vi "Alarm_TC_Cat.vi"() -> ()   [LabVIEW 2014]
panel:
  in  "T Target":dbl
  out "Error":u32
  in  "T Stoic":dbl
  out "Status Out":i32=300
  in  "Status In":i32=300
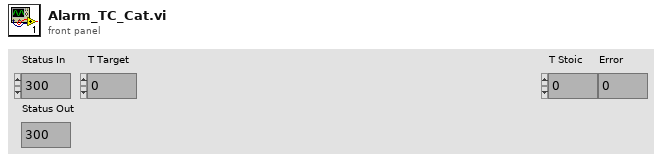
[diagram p1: front panel]
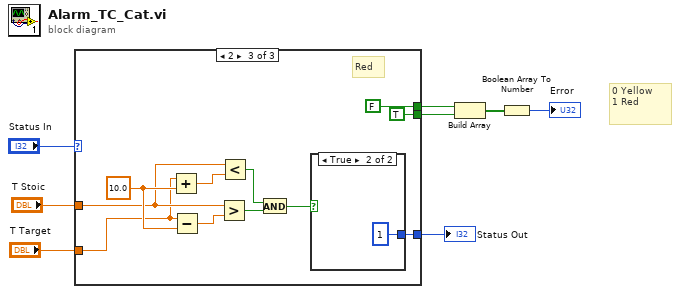
[diagram p0: block diagram]
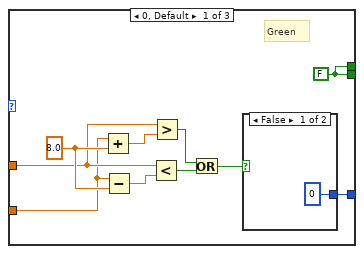
[diagram p2: hidden frame]
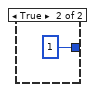
[diagram p3: hidden frame]
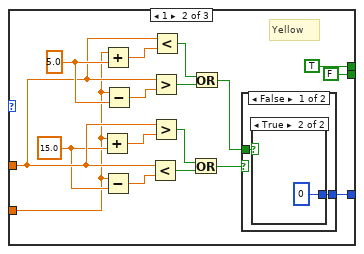
[diagram p4: hidden frame]
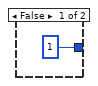
[diagram p5: hidden frame]
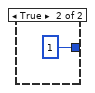
[diagram p6: hidden frame]
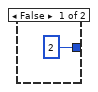
[diagram p7: hidden frame]
diagram:
  # "0 Yellow\n1 Red"
  n1 = case shown="2" "Status In" {
    tunnel: "T Stoic" -> [w11 w24 w47]
    tunnel: [w15 w32 w46] -> w6
    tunnel: [w10 TRUE ("x .or. y?") FALSE ("x .or. y?")] -> w5
    tunnel: [w10 FALSE ("x .or. y?") TRUE ("x .or. y?")] -> w4
    tunnel: "T Target" -> [w9 w21 w43]
    frame 0, Default {
      w10 = FALSE ("x .or. y?")
      w12 = 8.0 ("y")
      # "Green"
      n2 = Add(x=w9, y=w12) -> (x+y=w13:dbl)
      n3 = Subtract(x=w9, y=w12) -> (x-y=w14:dbl)
      n4 = Less?(x=w11, y=w14) -> (x < y?=w17:bool)
      n5 = Greater?(x=w11, y=w13) -> (0:w18:bool)
      n6 = Or(x=w18, y=w17) -> (x .or. y?=w16:bool)
      n7 = case shown="False" w16 {
        tunnel: [0 ("y") 1 ("y")] -> w15
        frame False {
        }
        frame True {
        }
      }
    }
    frame 1 {
      w25 = 5.0 ("y")
      w22 = 15.0 ("y")
      # "Yellow"
      n8 = Add(x=w21, y=w22) -> (x+y=w33:dbl)
      n9 = Add(x=w21, y=w25) -> (x+y=w26:dbl)
      n10 = Subtract(x=w21, y=w22) -> (x-y=w34:dbl)
      n11 = Subtract(x=w21, y=w25) -> (x-y=w27:dbl)
      n12 = Less?(x=w24, y=w34) -> (x < y?=w36:bool)
      n13 = Greater?(x=w24, y=w27) -> (0:w28:bool)
      n14 = Greater?(x=w24, y=w33) -> (0:w37:bool)
      n15 = Less?(x=w24, y=w26) -> (x < y?=w29:bool)
      n16 = Or(x=w37, y=w36) -> (x .or. y?=w35:bool)
      n17 = Or(x=w29, y=w28) -> (x .or. y?=w23:bool)
      n18 = case shown="False" w35 {
        tunnel: [w39 1 ("y")] -> w32
        tunnel: w23 -> [w38 _]
        frame False {
          n19 = case shown="True" w38 {
            tunnel: [1 ("y") 0 ("y")] -> w39
            frame False {
            }
            frame True {
            }
          }
        }
        frame True {
        }
      }
    }
    frame 2 {
      w48 = 10.0 ("y")
      # "Red"
      n20 = Add(x=w43, y=w48) -> (x+y=w49:dbl)
      n21 = Subtract(x=w43, y=w48) -> (x-y=w50:dbl)
      n22 = Greater?(x=w47, y=w50) -> (0:w52:bool)
      n23 = Less?(x=w47, y=w49) -> (x < y?=w53:bool)
      n24 = And(x=w53, y=w52) -> (x .and. y?=w51:bool)
      n25 = case shown="True" w51 {
        tunnel: [2 ("y") 1 ("y")] -> w46
        frame False {
        }
        frame True {
        }
      }
    }
  }
  "Status Out" <- w6
  n26 = Build Array(w5, w4) -> (w3:bool[])
  n27 = Boolean Array To Number(Boolean array=w3) -> (number=→"Error":u32)
